vi "Do.vi"(8 "error in (no error)":errorcluster, 10 "Actor in":refnum<class "Actor.lvclass">, 11 "Register Variant Msg":refnum<class "Register Project Number Msg.lvclass">) -> (0 "error out":errorcluster, 2 "Actor out":refnum<class "Actor.lvclass">)   [LabVIEW 2013, in "Main Model.lvlib" / "Register Project Number Msg.lvclass"]
doc: "(<B>Filename</B>: Actor Framework.lvlib:Message.lvclass:Do.vi)\n\nDefines what a message does when it is received by an actor. Generally, a message instructs an actor to invoke one of its methods.\n\nBy default, this method does nothing. A child class must override it to define behavior. Create a child class by using the Actor Framework Message Maker dialog box."
uses:
  Register Project Number Msg.lvclass
  <vilib>/ActorFramework/Actor/Actor.lvclass
  Main Model/Main Model.lvclass
  <vilib>/ActorFrameworkMVC/View Observer/Registration Message/Registration Message.lvclass/Registration Message.ctl
  <vilib>/ActorFramework/Message Enqueuer/Message Enqueuer.lvclass
  <vilib>/ActorFrameworkMVC/View Observer/Data Message/Data Message.lvclass
  <vilib>/ActorFrameworkMVC/View Observer/Registration Message/Registration Message.lvclass
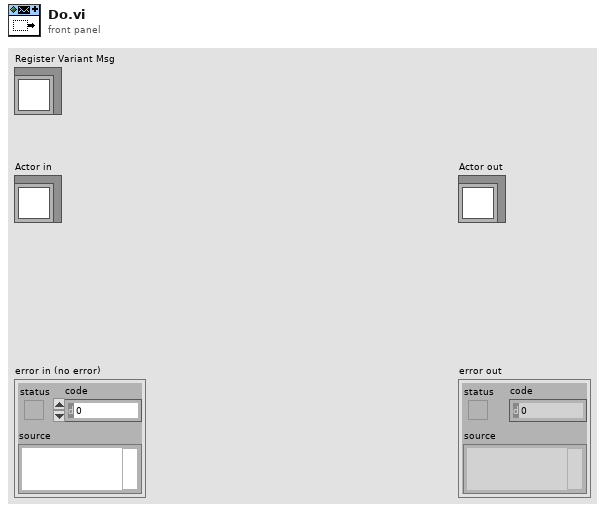
[diagram p1: front panel]
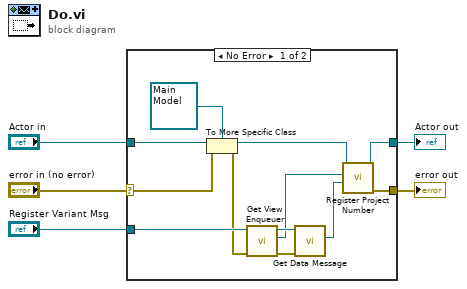
[diagram p0: block diagram]
diagram:
  n1 = case shown="No Error" "error in (no error)" {
    selector: "error in (no error)" -> [w7 w19]
    tunnel: "Register Variant Msg" -> [w16 _]
    tunnel: "Actor in" -> [w15 w18]
    tunnel: [w12 w18] -> w3
    tunnel: [w8 w19] -> w2
    frame No Error {
      n2 = To More Specific Class(target class=refnum<class "Main Model.lvclass"> refnum ("Model Actor.lvlib:Model Actor.lvclass"), reference=w15, error in=w7) -> (specific class reference=w13:refnum<class "Main Model.lvclass">, error out=w6:errorcluster)
      n3 = call <vilib>:"Get View Enqueuer.vi"("error in (no error)"=w6, "Registration Message in"=w16) -> ("error out"=w11:errorcluster, "View Enqueuer"=w10:refnum<class "Message Enqueuer.lvclass">, "Registration Message out"=w17:refnum<class "Register Project Number Msg.lvclass">)  [unwired: 7 in]
      n4 = call <vilib>:"Get Data Message.vi"("error in (no error)"=w11, "Registration Message in"=w17) -> ("Data Message"=w9:refnum<class "Data Message.lvclass">)  [unwired: 7 in, 2 out]
      n5 = call "Register Project Number.vi"("Data Message"=w9, "View Enqueuer"=w10, "Main Model in"=w13) -> ("error out"=w8:errorcluster, "Main Model out"=w12:refnum<class "Main Model.lvclass">)  [unwired: 7 in]
    }
    frame Error {
    }
  }
  "error out" <- w2
  "Actor out" <- w3
